vi "Control Experiment FGV.vi"(6 "Function":enum16{"read", "write"}(ring), 8 "error in (no error)":errorcluster, 11 "Control Experiment":refnum<class "SMO.Control Experiment.lvclass">) -> (0 "error out":errorcluster, 3 "Control Experiment out":refnum<class "SMO.Control Experiment.lvclass">)   [LabVIEW 2019, in "SMO.Control Experiment.lvclass"]
uses:
  SMO.Control Experiment.lvclass
  <vilib>/Utility/sysdir.llb/System Directory Type.ctl
  <vilib>/Utility/xml.llb/Read From XML File(string).vi
  <vilib>/Utility/xml.llb/Write to XML File(string).vi
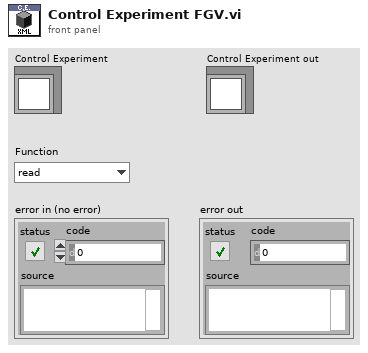
[diagram p1: front panel]
types:
  T1 = typedef "System Directory Type.ctl" = i32
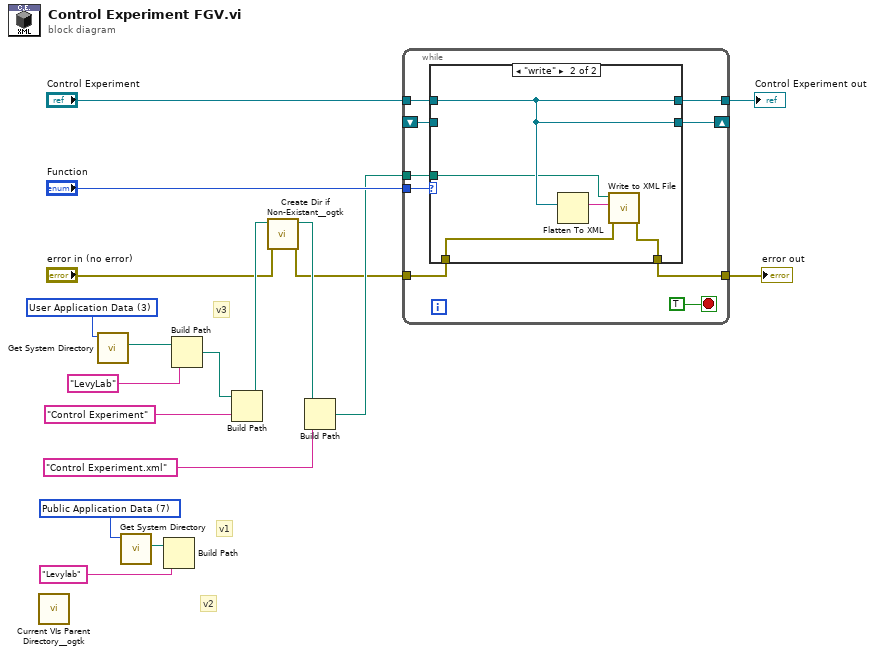
[diagram p0: block diagram]
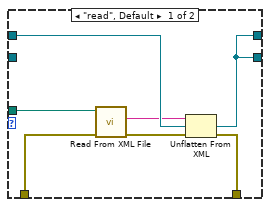
[diagram p2: hidden frame]
diagram:
  w8 = T1 3 items=["User Home"=0, "User Desktop"=1, "User Documents"=2, "User Application Data"=3, "User Preferences"=4, "User Temporary"=5, "Public Documents"=6, "Public Application Data"=7, "Public Preferences"=8, "Public Cache"=13, "System Core Libraries"=9, "System Installed Libraries"=10, "Application Files"=11, "Boot Volume Root"=12] ("system directory type")
  w13 = T1 7 items=["User Home"=0, "User Desktop"=1, "User Documents"=2, "User Application Data"=3, "User Preferences"=4, "User Temporary"=5, "Public Documents"=6, "Public Application Data"=7, "Public Preferences"=8, "Public Cache"=13, "System Core Libraries"=9, "System Installed Libraries"=10, "Application Files"=11, "Boot Volume Root"=12] ("system directory type")
  # "v3"
  # "v2"
  # "v1"
  n1 = call <userlib>:"Current VIs Parent Directory__ogtk.vi"() -> ()  [unwired: 5 in, 1 out]
  n2 = call <vilib>:"Get System Directory.vi"("system directory type"=w8) -> ("system directory"=w7:path)  [unwired: 10 in]
  n3 = call <vilib>:"Get System Directory.vi"("system directory type"=w13) -> ("system directory"=w11:path)  [unwired: 10 in]
  n4 = Build Path(base path=w11, name or relative path="Levylab") -> ()  [unwired: 1 out]
  n5 = Build Path(base path=w7, name or relative path="LevyLab") -> (appended path=w5:path)
  n6 = Build Path(base path=w5, name or relative path="Control Experiment") -> (appended path=w4:path)
  n7 = call <userlib>:"Create Dir if Non-Existant__ogtk.vi"("error in (no error)"="error in (no error)", "Directory Path"=w4) -> ("error out"=w1:errorcluster, "dup Directory Path"=w3:path)  [unwired: 7 in, 1 out]
  n8 = Build Path(base path=w3, name or relative path="Control Experiment.xml") -> (appended path=w9:path)
  n9 = while {
    tunnel: "Control Experiment" -> [w24]
    tunnel: w1 -> [w21]
    tunnel: [w20] -> w18
    tunnel: [w23] -> w15
    shift-right: [w25] -> _
    shift-left: _ -> [w22]
    tunnel: "Function" -> [w26]
    tunnel: w9 -> [w19]
    stop <- TRUE stop-if-true
    n10 = case shown="\"write\"" w26 {
      tunnel: [w33 w39] -> w25
      tunnel: w24 -> [w32 w39]
      tunnel: [w33 w39] -> w23
      tunnel: w22 -> [_ _]
      tunnel: w21 -> [w29 w38]
      tunnel: [w34 w35] -> w20
      tunnel: w19 -> [w31 w36]
      frame "read", Default {
        n11 = call-poly <vilib>:"Read From XML File.vi"("error in (no error)"=w29, "XML File Path"=w31) -> ("error out"=w28:errorcluster, "XML Elements"=w30:string)  [unwired: 7 in, 1 out]
        n12 = Unflatten From XML(xml string=w30, type=w32, error in (no error)=w28) -> (value=w33:refnum<class "SMO.Control Experiment.lvclass">, error out=w34:errorcluster)
      }
      frame "write" {
        n13 = Flatten To XML(anything=w39) -> (xml string=w37:string)
        n14 = call-poly <vilib>:"Write to XML File.vi"("error in (no error)"=w38, "XML Input"=w37, "XML File Path"=w36) -> ("error out"=w35:errorcluster)  [unwired: 6 in, 2 out]
      }
    }
  }
  "error out" <- w18
  "Control Experiment out" <- w15
